vi "Greatest_Common_Factor.vi"() -> ()   [LabVIEW 2022 SP3]
panel:
  out "Greatest Common Factor":dbl
  in  "B":dbl
  in  "A":dbl
  # "Greatest_Common_Factor:\nEnter any 2 integers, A and B, to find their\ngreatest common factor. This is done using \nEuclid's method. If 1 is the only common factor,\nyou will be notified of this."
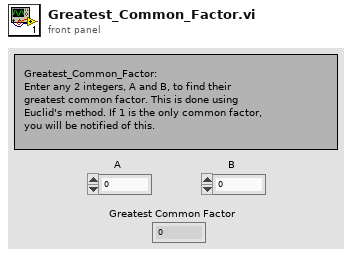
[diagram p1: front panel]
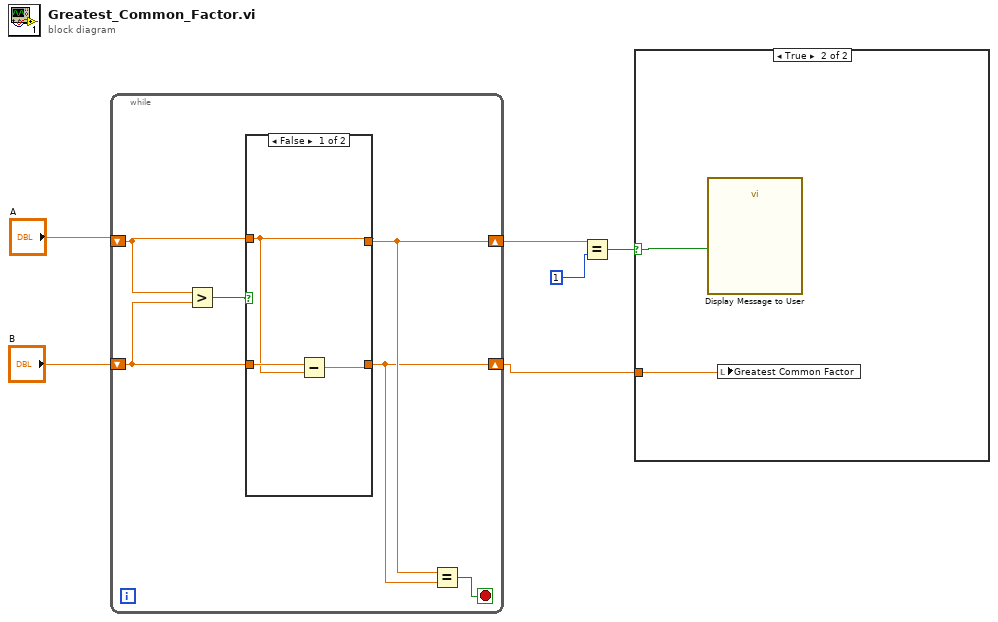
[diagram p0: block diagram]
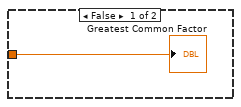
[diagram p2: hidden frame]
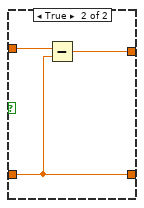
[diagram p3: hidden frame]
diagram:
  n1 = while {
    shift-right: [w8] -> w4
    shift-left: "A" -> [w11]
    shift-right: [w7] -> w1
    shift-left: "B" -> [w10]
    stop <- w9 stop-if-true
    n2 = Greater?(x=w11, y=w10) -> (0:w12:bool)
    n3 = case shown="False" w12 {
      tunnel: w11 -> [w13 w18]
      tunnel: w10 -> [w15 w16]
      tunnel: [w13 w17] -> w8
      tunnel: [w14 w16] -> w7
      frame False {
        n4 = Subtract(x=w15, y=w13) -> (x-y=w14:dbl)
      }
      frame True {
        n5 = Subtract(x=w18, y=w16) -> (x-y=w17:dbl)
      }
    }
    n6 = Equal?(x=w8, y=w7) -> (x = y?=w9:bool)
  }
  n7 = Equal?(x=w4, y=1) -> (x = y?=w2:bool)
  n8 = case shown="True" w2 {
    selector: w2 -> [_ w21]
    tunnel: w1 -> [w19 w20]
    frame False {
      "Greatest Common Factor" <- w19
    }
    frame True {
      n9 = call "Display Message to User"("Enable"=w21) -> ()  [unwired: 9 in, 2 out]
      n10 = local write "Greatest Common Factor"(w20) -> ()
    }
  }
